vi "CMD_Harvest.vi"(1 "Line":string) -> (0 "Done":bool)   [LabVIEW 2017, in "Apple script.lvlib"]
uses:
  Apple script.lvlib
  Robot Global Data.vi
panel:
  in  "Parameters":i32[](array[numeric])=[1, 1, 0]
  in  "Subcommands":string[](array[string])=["for", "at", "stop"]
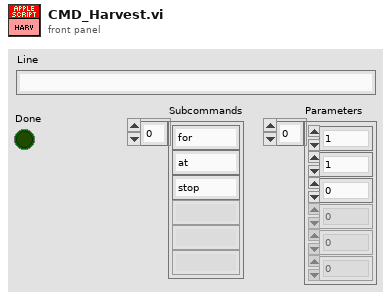
[diagram p1: front panel]
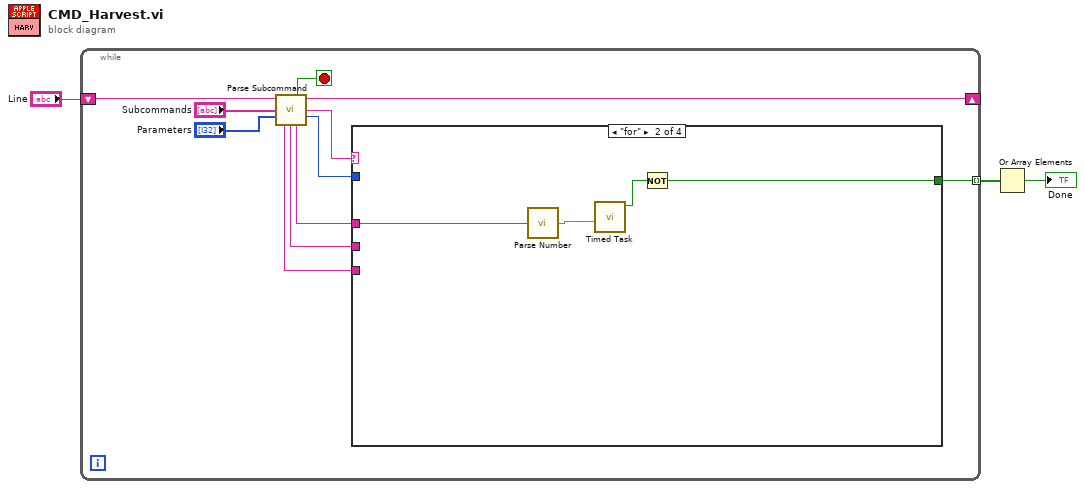
[diagram p0: block diagram]
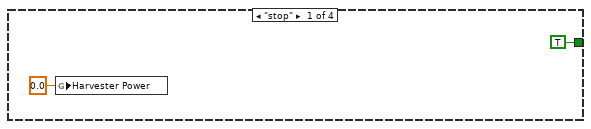
[diagram p2: hidden frame]
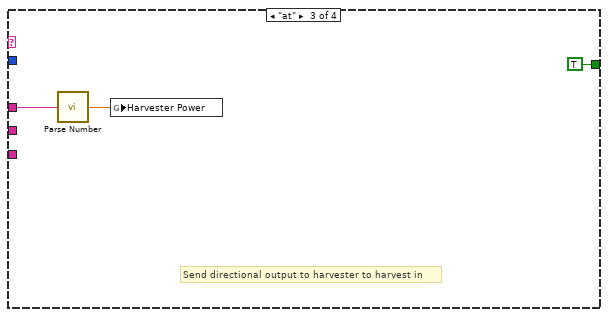
[diagram p3: hidden frame]
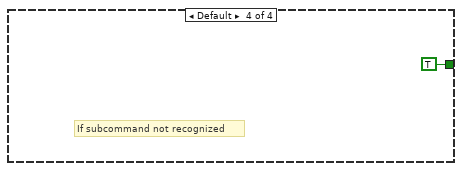
[diagram p4: hidden frame]
diagram:
  n1 = while {
    shift-right: [w11] -> _
    shift-left: "Line" -> [w14]
    tunnel: [w4] -> w2 mode=indexing
    stop <- w10 stop-if-true
    n2 = call "Parse Subcommand.vi"("Text In"=w14, "Subcommands"="Subcommands", "Parameters"="Parameters") -> ("Done"=w10:bool, "Text Out"=w11:string, "Subcommand"=w9:string, "# of Parameters"=w8:i32, "Parameter 3"=w5:string, "Parameter 2"=w6:string, "Parameter 1"=w7:string)  [unwired: 6 in]
    n3 = case shown="\"for\"" w9 {
      tunnel: w8 -> [_ _ _ _]
      tunnel: w7 -> [_ w19 w22 _]
      tunnel: w6 -> [_ _ _ _]
      tunnel: w5 -> [_ _ _ _]
      tunnel: [TRUE ("Done") w17 TRUE ("Done") TRUE] -> w4
      frame "stop" {
        n4 = global write "Robot Global Data.vi" "Harvester Power"(0.0 ("Harvester Power")) -> ()
      }
      frame "for" {
        n5 = call "Parse Number.vi"("String"=w19) -> ("Number"=w20:dbl)
        n6 = call "Timed Task.vi"("Time (ms)"=w20) -> ("Running"=w18:bool)  [unwired: 10 in]
        n7 = Not(x=w18) -> (.not. x?=w17:bool)
      }
      frame "at" {
        # "Send directional output to harvester to harvest in"
        n8 = call "Parse Number.vi"("String"=w22) -> ("Number"=w21:dbl)
        n9 = global write "Robot Global Data.vi" "Harvester Power"(w21) -> ()
      }
      frame Default {
        # "If subcommand not recognized"
      }
    }
  }
  n10 = Or Array Elements(Boolean array=w2) -> (logical OR=→"Done":bool)
